vi "estadoTorre.vi"(2 "¿pieza?":i32, 3 "estadoTorre":i8[](array[numeric])) -> (0 "¿disponible?":bool, 1 "posicionCero":i32)   [LabVIEW 2020]
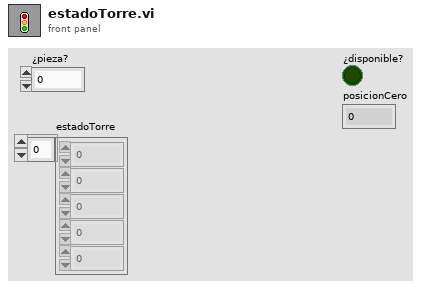
[diagram p1: front panel]
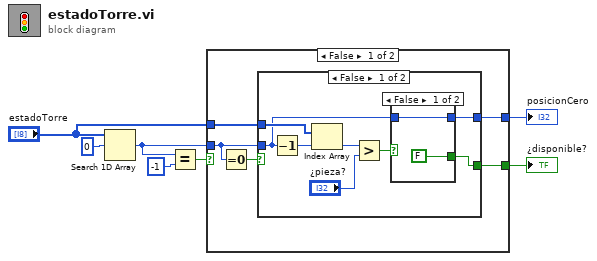
[diagram p0: block diagram]
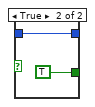
[diagram p2: hidden frame]
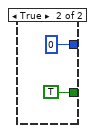
[diagram p3: hidden frame]
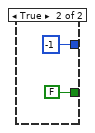
[diagram p4: hidden frame]
diagram:
  n1 = Search 1D Array(1D array="estadoTorre", element=i8 0) -> (index of element=w3:i32)  [unwired: 1 in]
  n2 = Equal?(x=w3, y=-1) -> (x = y?=w5:bool)
  n3 = case shown="False" w5 {
    tunnel: [w11 FALSE] -> w1
    tunnel: [w10 -1] -> w2
    tunnel: "estadoTorre" -> [w9 _]
    tunnel: w3 -> [w8 _]
    frame False {
      n4 = Equal To 0?(x=w8) -> (x = 0?=w12:bool)
      n5 = case shown="False" w12 {
        tunnel: [w15 TRUE] -> w11
        tunnel: [w13 0] -> w10
        tunnel: w9 -> [w20 _]
        tunnel: w8 -> [w14 _]
        frame False {
          n6 = Decrement(x=w14) -> (x-1=w19:i32)
          n7 = Index Array(array=w20, index=w19) -> (element=w18:i8)
          n8 = Greater?(x=w18, y="¿pieza?") -> (0:w16:bool)
          n9 = case shown="False" w16 {
            tunnel: [FALSE TRUE] -> w15
            tunnel: w14 -> [w21 w23]
            tunnel: [w21 w23] -> w13
            frame False {
            }
            frame True {
            }
          }
        }
        frame True {
        }
      }
    }
    frame True {
    }
  }
  "posicionCero" <- w2
  "¿disponible?" <- w1
